vi "SSC DCPower Configure and Start Waveform Acquisition.vi"(0 "DCPower SSC in":T3[](array[typedef]), 5 "Sample Rate (Hz)":dbl=inf caption="Sample Rate (Max Hz)" format="%#_6p", 7 "Buffer Length (s)":dbl=1.0 caption="Buffer Length (1 second)" format="%#_6p", 11 "error in":errorcluster) -> (3 "Settings":T1 {"Previous Settings"."Triggers:Measure Trigger:Trigger Type" items=["Digital Edge"=1014, "Software Edge"=1015, "None"=1012]; "Previous Settings"."Measurement:Advanced:Measure When" items=["Automatically after Source Complete"=1025, "On Demand"=1026, "On Measure Trigger"=1027]; "Previous Settings"."Measurement:Aperture Time" format="%#_6p"; "Previous Settings"."Measurement:Aperture Time Units" items=["Seconds"=1028, "Power Line Cycles"=1029]}, 4 "DCPower SSC out":T3[](array[typedef]), 15 "error out":errorcluster)   [LabVIEW 2020]
doc: "This VI aborts the task, configures the tasks for waveform acquisition, initializes the task and starts the acquisition."
uses:
  SSC DCPower.ctl
  SSC DCPower Waveform Acquisition Saved Settings.ctl
  SSC DCPower Waveform Acquisition Saved Setting.ctl
  <instrlib>/niDCPower/nidcpower.llb/niDCPower Send Software Edge Trigger - Signal.ctl
  <instrlib>/niDCPower/nidcpower.llb/niDCPower Send Software Edge Trigger.vi
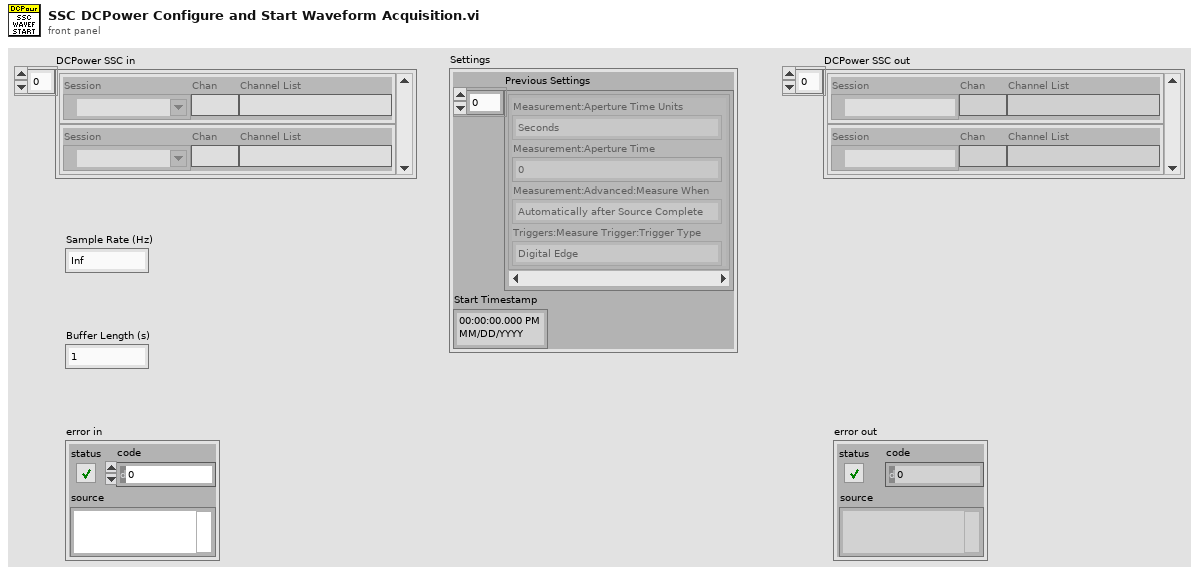
[diagram p1: front panel]
types:
  T1 = typedef "SSC DCPower Waveform Acquisition Saved Settings.ctl" = cluster{"Previous Settings":T2[], "Start Timestamp":timestamp}
  T2 = typedef "SSC DCPower Waveform Acquisition Saved Setting.ctl" = cluster{"Measurement:Aperture Time Units":i32, "Measurement:Aperture Time":dbl, "Measurement:Advanced:Measure When":i32, "Triggers:Measure Trigger:Trigger Type":i32}
  T3 = typedef "SSC DCPower.ctl" = cluster{"Session":refnum<k15>, "Chan":string, "Channel List":string}
  T4 = typedef "niDCPower Send Software Edge Trigger - Signal.ctl" = i32
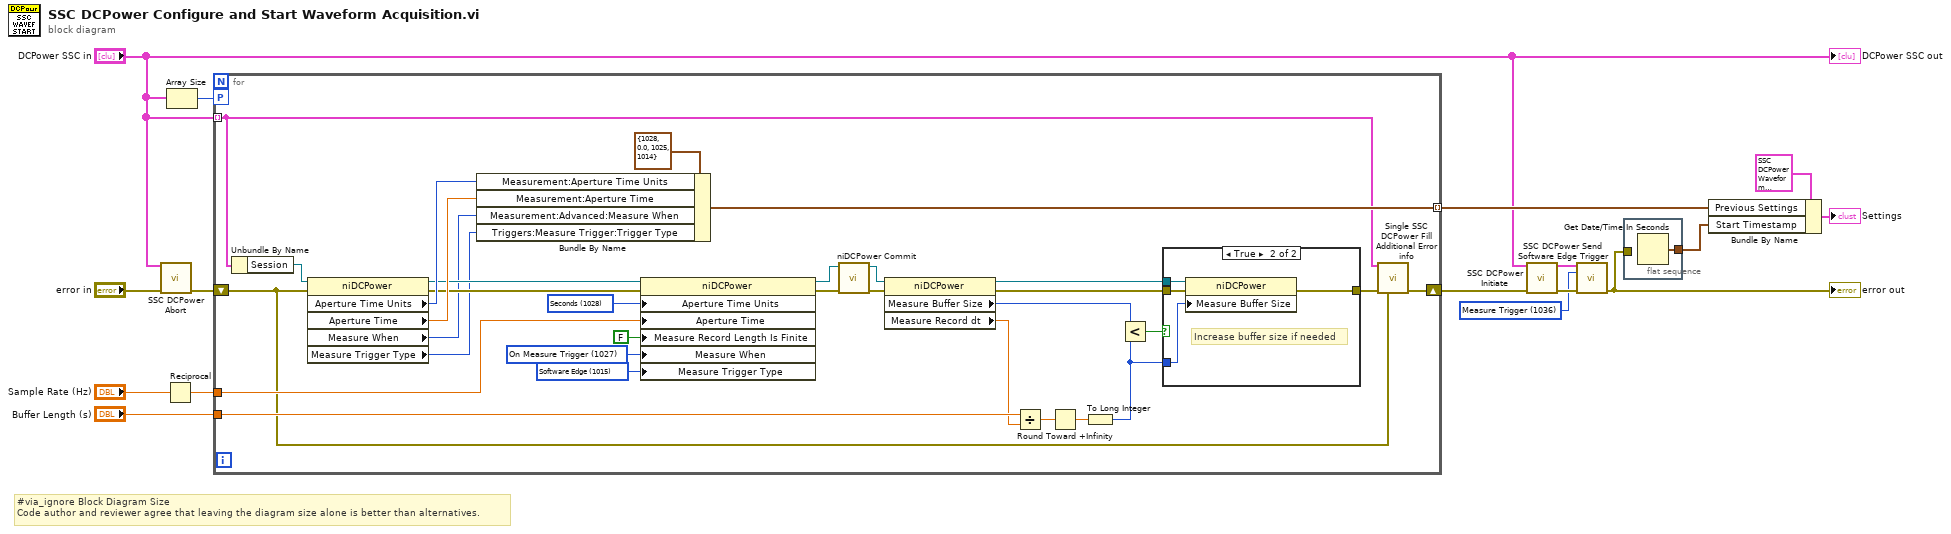
[diagram p0: block diagram]
diagram:
  w6 = T4 1036 items=["Start Trigger"=1034, "Source Trigger"=1035, "Measure Trigger"=1036, "Sequence Advance Trigger"=1037, "Pulse Trigger"=1053] ("Trigger to Send")
  # "#via_ignore Block Diagram Size\nCode author and reviewer agree that leaving the diagram size alone is better than alternatives."
  n1 = call "SSC DCPower Abort.vi"("DCPower SSC in"="DCPower SSC in", "error in"="error in") -> ("error out"=w14:errorcluster)  [unwired: 12 in, 1 out]
  n2 = Reciprocal(x="Sample Rate (Hz)") -> (1/x=w12:dbl)
  n3 = Array Size(array="DCPower SSC in") -> (size(s)=w4:i32)
  n4 = for {
    tunnel: "DCPower SSC in" -> [w18] mode=indexing
    workers-P: w4 -> [_]
    tunnel: w12 -> [w47]
    tunnel: [w46] -> w10 mode=indexing
    shift-right: [w19] -> w5
    shift-left: w14 -> [w17]
    tunnel: "Buffer Length (s)" -> [w26]
    w37 = 1015 items=["Digital Edge"=1014, "Software Edge"=1015, "None"=1012] ("Triggers:Measure Trigger:Trigger Type")
    w38 = 1027 items=["Automatically after Source Complete"=1025, "On Demand"=1026, "On Measure Trigger"=1027] ("Measurement:Advanced:Measure When")
    w40 = 1028 items=["Seconds"=1028, "Power Line Cycles"=1029] ("Measurement:Aperture Time Units")
    n5 = Unbundle By Name(w18) -> ("Session"=w45:refnum<k15>)
    n6 = property class="niDCPower"(reference=w45, error in=w17) -> (reference out=w41:refnum<k15>, error out=w42:errorcluster, "Aperture Time Units"=w44:i32, "Aperture Time"=w43:dbl, "Measure When"=w36:i32, "Measure Trigger Type"=w35:i32)
    n7 = Bundle By Name(cluster=T2 {"Measurement:Aperture Time Units"=1028, "Measurement:Aperture Time"=0.0, "Measurement:Advanced:Measure When"=1025, "Triggers:Measure Trigger:Trigger Type"=1014} ("Settings"), "Measurement:Aperture Time Units"=w44, "Measurement:Aperture Time"=w43, "Measurement:Advanced:Measure When"=w36, "Triggers:Measure Trigger:Trigger Type"=w35) -> (w46:T2)
    n8 = property class="niDCPower"(reference=w41, error in=w42, "Aperture Time Units"=w40, "Aperture Time"=w47, "Measure Record Length Is Finite"=FALSE ("Measurement:Measure Record Length Is Finite"), "Measure When"=w38, "Measure Trigger Type"=w37) -> (reference out=w31:refnum<k15>, error out=w32:errorcluster)
    n9 = call <instrlib>:"niDCPower Commit.vi"("error in (no error)"=w32, "instrument handle"=w31) -> ("error out"=w33:errorcluster, "instrument handle out"=w29:refnum<k15>)  [unwired: 8 in]
    n10 = property class="niDCPower"(reference=w29, error in=w33) -> (reference out=w27:refnum<k15>, error out=w30:errorcluster, "Measure Buffer Size"=w22:i32, "Measure Record dt"=w25:dbl)
    n11 = Divide(x=w26, y=w25) -> (x/y=w24:dbl)
    n12 = Round Toward +Infinity(x=w24) -> (ceil(x): smallest int >= x=w23:dbl)
    n13 = To Long Integer(number=w23) -> (32bit integer=w20:i32)
    n14 = Less?(x=w22, y=w20) -> (x < y?=w21:bool)
    n15 = case shown="True" w21 {
      tunnel: w30 -> [w48 w52]
      tunnel: [w48 w51] -> w28
      tunnel: w27 -> [_ w50]
      tunnel: w20 -> [_ w49]
      frame False {
      }
      frame True {
        # "Increase buffer size if needed"
        n16 = property class="niDCPower"(reference=w50, error in=w52, "Measure Buffer Size"=w49) -> (error out=w51:errorcluster)  [unwired: 1 out]
      }
    }
    n17 = call "Single SSC DCPower Fill Additional Error info.vi"("DCPower SSC in"=w18, "error in"=w28, "previous error in"=w17) -> ("error out"=w19:errorcluster)  [unwired: 12 in]
  }
  n18 = call "SSC DCPower Initiate.vi"("DCPower SSC in"="DCPower SSC in", "error in"=w5) -> ("DCPower SSC out"=w3:T3[], "error out"=w16:errorcluster)  [unwired: 12 in]
  n19 = call "SSC DCPower Send Software Edge Trigger.vi"("DCPower SSC in"=w3, "Trigger to Send"=w6, "error in"=w16) -> ("error out"=w11:errorcluster)  [unwired: 11 in, 1 out]
  "error out" <- w11
  n20 = flat-sequence {
    tunnel: [w53] -> w9
    tunnel: w11 -> [_]
    frame #0 {
      n21 = Get Date/Time In Seconds() -> (seconds since 1Jan1904=w53:timestamp)
    }
  }
  n22 = Bundle By Name(cluster=T1 {"Previous Settings"=[], "Start Timestamp"=timestamp(0 s since 1904-01-01)} ("Settings"), "Previous Settings"=w10, "Start Timestamp"=w9) -> (→"Settings":T1)
  "DCPower SSC out" <- "DCPower SSC in"
